vi "Fired.vi"(8 "error in (no error)":errorcluster, 9 "Hit Targets":string[](array[string]), 10 "World In":refnum<class "3D Object.lvclass">, 11 "Player in":refnum<class "Player.lvclass">) -> (0 "error out":errorcluster, 3 "Player out":refnum<class "Player.lvclass">)   [LabVIEW 2015, in "Player.lvclass"]
uses:
  Player.lvclass
  3D Object/3D Object.lvclass
  Player.lvclass/Player.ctl
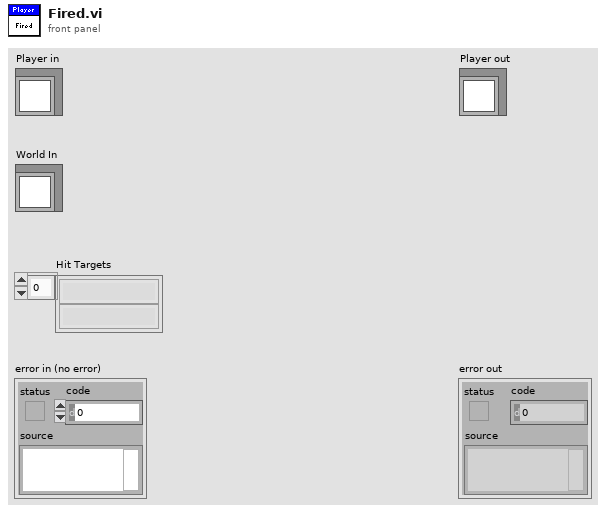
[diagram p1: front panel]
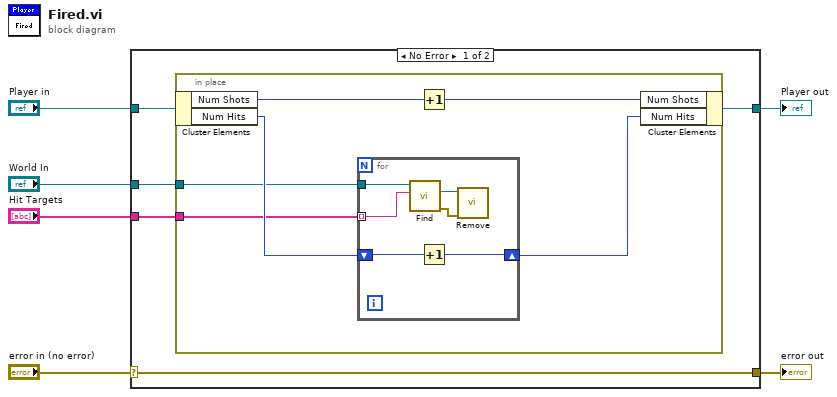
[diagram p0: block diagram]
diagram:
  n1 = case shown="No Error" "error in (no error)" {
    selector: "error in (no error)" -> [w11 w25]
    tunnel: [w11 w25] -> w5
    tunnel: [w9 w24] -> w3
    tunnel: "Player in" -> [w10 w24]
    tunnel: "Hit Targets" -> [w8 _]
    tunnel: "World In" -> [w7 _]
    frame No Error {
      n2 = in-place {
        in-place-border: w8 -> [w13]
        in-place-border: w7 -> [w12]
        n3 = in-place-cluster #1(w10) -> ("Num Shots"=w17:i32, "Num Hits"=w15:i32)
        n4 = for {
          shift-right: [w22] -> w14
          shift-left: w15 -> [w23]
          tunnel: w13 -> [w21] mode=indexing
          tunnel: w12 -> [w20]
          n5 = call "Find.vi"("Name"=w21, "World In"=w20) -> ("error out"=w18:errorcluster, "Object out"=w19:refnum<class "3D Object.lvclass">)  [unwired: 7 in, 1 out]
          n6 = Increment(x=w23) -> (x+1=w22:i32)
          n7 = call "Remove.vi"("error in (no error)"=w18, "3D Object in"=w19) -> ()  [unwired: 9 in, 1 out]
        }
        n8 = Increment(x=w17) -> (x+1=w16:i32)
        n9 = in-place-cluster #1("Num Shots"=w16, "Num Hits"=w14) -> (w9:refnum<class "Player.lvclass">)
      }
    }
    frame Error {
    }
  }
  "error out" <- w5
  "Player out" <- w3
